vi "create.vi"(8 "error in (no error)":errorcluster, 10 "Month":refnum<vi>, 11 "Year":refnum<vi>) -> (0 "error out":errorcluster, 3 "MonthDisplay out":refnum<class "DateUserInterface.lvclass">)   [LabVIEW 2018, in "DateUserInterface.lvclass"]
uses:
  DateUserInterface.lvclass
  month.ctl
  DateUserInterface.lvclass/DateUserInterface.ctl
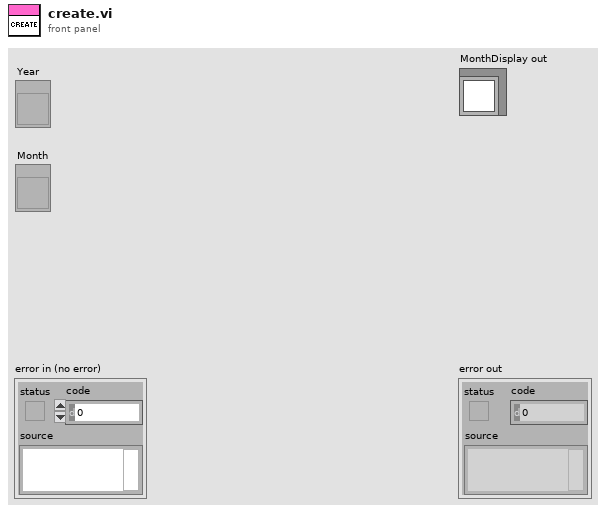
[diagram p1: front panel]
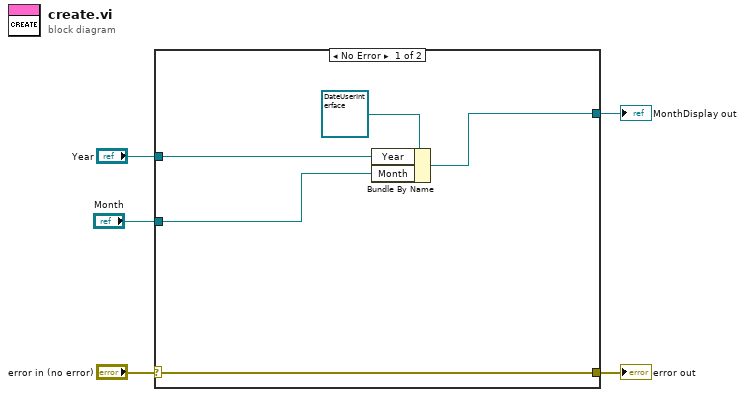
[diagram p0: block diagram]
diagram:
  n1 = case shown="No Error" "error in (no error)" {
    selector: "error in (no error)" -> [w10 w11]
    tunnel: [w10 w11] -> w4
    tunnel: [w6 _] -> w3
    tunnel: "Year" -> [w8 _]
    tunnel: "Month" -> [w7 _]
    frame No Error {
      n2 = Bundle By Name(cluster=refnum<class "DateUserInterface.lvclass"> refnum ("MonthDisplay.lvclass"), "Year"=w8, "Month"=w7) -> (w6:refnum<class "DateUserInterface.lvclass">)
    }
    frame Error {
    }
  }
  "error out" <- w4
  "MonthDisplay out" <- w3
